vi "ActorDatabase-PerformQuery.vi"(8 "error in (no error)":errorcluster, 10 "Payload from Actor":string, 11 "Database-Actor in":refnum<class "PartCertDatabase-Actor.lvclass">) -> (0 "error out":errorcluster, 2 "Payload To Actor":string, 3 "Database-Actor out":refnum<class "PartCertDatabase-Actor.lvclass">)   [LabVIEW 2013, in "PartCertDatabase-Actor.lvclass"]
uses:
  PartCertDatabase-Actor.lvclass
  PartCertDatabase-Actor.lvclass/PartCertDatabase-Actor.ctl
  ftw-dataflow/Core/src/Reflection/FTW-Reflection-Type.vi
  ftw-dataflow/Core/src/JSON/FTW-JSON-Core-LibraryFilepath.vi
  ftw-dataflow/Core/src/JSON/FTW-JSON-Core-GetFlattenedValue.vi
  ftw-dataflow/Core/src/JSON/FTW-JSON-Core-LibraryError.vi
  ftw-dataflow/Core/utils/CodeGen/JSON Deserialize/FTW-JSON-Deserialize.xnode
  Reuse Library/Database API/PartCertDatabase-API.lvclass
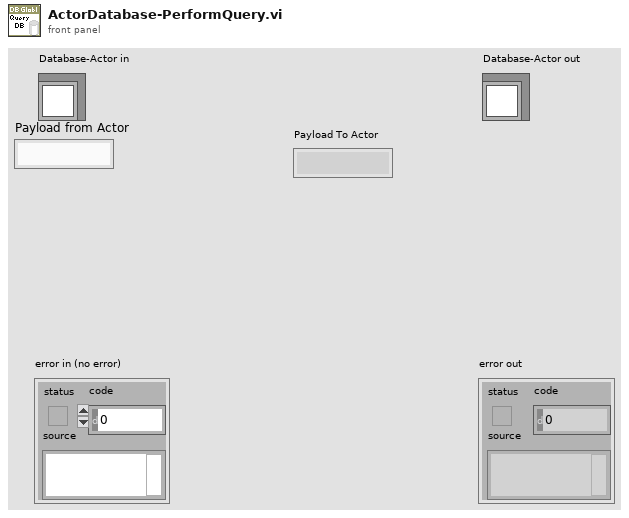
[diagram p1: front panel]
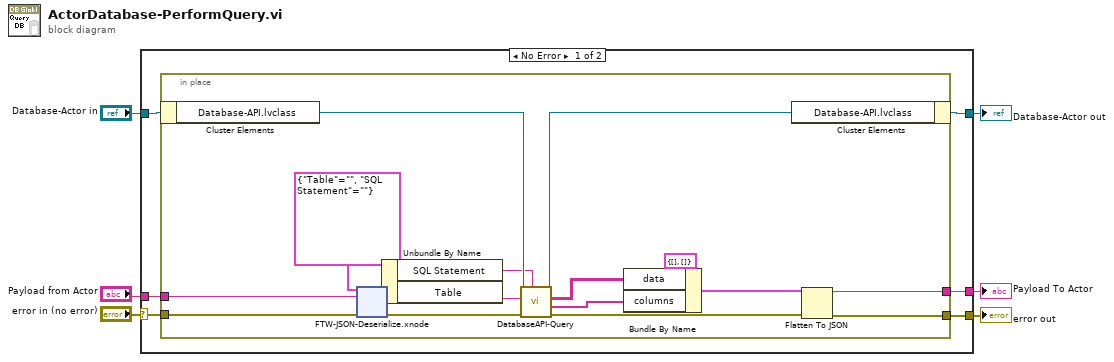
[diagram p0: block diagram]
diagram:
  n1 = case shown="No Error" "error in (no error)" {
    selector: "error in (no error)" -> [w12 w64]
    tunnel: [w11 w64] -> w5
    tunnel: [w9 w63] -> w3
    tunnel: "Database-Actor in" -> [w10 w63]
    tunnel: [w8 _] -> w2
    tunnel: "Payload from Actor" -> [w7 _]
    frame No Error {
      n2 = in-place {
        in-place-border: w12 -> [w20]
        in-place-border: [w19] -> w11
        in-place-border: [w18] -> w8
        in-place-border: w7 -> [w13]
        n3 = in-place-cluster #1(w10) -> ("Database-API.lvclass"=w28:refnum<class "PartCertDatabase-API.lvclass">)
        n4 = xnode "FTW-JSON-Deserialize.xnode"("Type and Defaults"=cluster{"Table":string, "SQL Statement":string} {"Table"="", "SQL Statement"=""}, "JSON String"=w13, "error in"=w20) -> ("Values"=w16:cluster{"Table":string, "SQL Statement":string}, "error out"=w27:errorcluster)
        n5 = Unbundle By Name(w16) -> ("SQL Statement"=w25:string, "Table"=w26:string)
        n6 = call "DatabaseAPI-Query.vi"("optional clause"=w25, "error in (no error)"=w27, "Table"=w26, "Database-API in"=w28) -> ("error out"=w21:errorcluster, "columns"=w14:string[], "data"=w15:string[][], "Database-API out"=w24:refnum<class "PartCertDatabase-API.lvclass">)  [unwired: 4 in]
        n7 = Bundle By Name(cluster=cluster{"data":string[][], "columns":string[]} {"data"=[], "columns"=[]}, "data"=w15, "columns"=w14) -> (w22:cluster{"data":string[][], "columns":string[]})
        n8 = in-place-cluster #1("Database-API.lvclass"=w24) -> (w9:refnum<class "PartCertDatabase-Actor.lvclass">)
        n9 = Flatten To JSON(anything=w22, error in (no error)=w21) -> (JSON string=w18:string, 11:w19:errorcluster)  [unwired: 1 in]
      }
    }
    frame Error {
    }
  }
  "error out" <- w5
  "Database-Actor out" <- w3
  "Payload To Actor" <- w2
